vi "getConfigurationConnectionInfo.vi"(8 "error in (no error)":errorcluster, 11 "IDeviceInfo in":refnum<class "IDeviceInfo.lvclass">) -> (0 "error out":errorcluster, 2 "DeviceType out":refnum<class "IServerCapability.lvclass">, 3 "IDeviceInfo out":refnum<class "IDeviceInfo.lvclass">)   [LabVIEW 2022 SP3, in "openDAQ.lvlib" / "IBaseObject.lvlib" / "IPropertyObject.lvlib" / "IDeviceInfo.lvlib" / "IDeviceInfo.lvclass"]
uses:
  <instrlib>/openDAQ/Public/Classes/IDeviceInfo/IDeviceInfo.lvclass
  <instrlib>/openDAQ/Public/Classes/IDeviceInfo/IDeviceInfo.lvclass/IDeviceInfo.ctl
  <instrlib>/openDAQ/Binaries/Windows/x86/copendaq32.dll
  <instrlib>/openDAQ/Public/Classes/IServerCapability/IServerCapability.lvclass
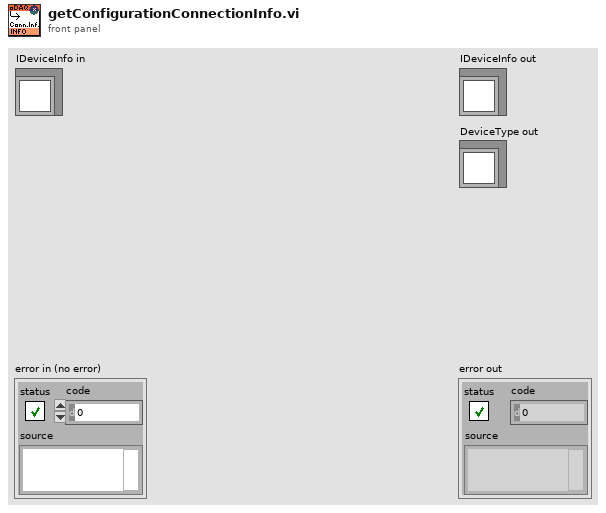
[diagram p1: front panel]
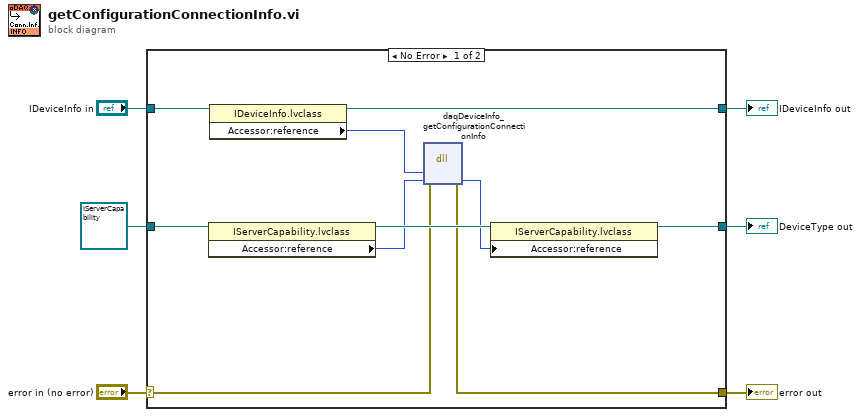
[diagram p0: block diagram]
diagram:
  n1 = case shown="No Error" "error in (no error)" {
    selector: "error in (no error)" -> [w9 w18]
    tunnel: [w7 w18] -> w5
    tunnel: [w13 w17] -> w3
    tunnel: "IDeviceInfo in" -> [w15 w17]
    tunnel: refnum<class "IServerCapability.lvclass"> refnum -> [w10 _]
    tunnel: [w8 _] -> w1
    frame No Error {
      n2 = property class="IServerCapability.lvclass"(reference=w10) -> (reference out=w16:refnum<class "IServerCapability.lvclass">, "Accessor:reference"=w12:i64)  [unwired: 1 in, 1 out]
      n3 = property class="IDeviceInfo.lvclass"(reference=w15) -> (reference out=w13:refnum<class "IDeviceInfo.lvclass">, "Accessor:reference"=w14:i64)  [unwired: 1 in, 1 out]
      n4 = dll-call lib="C:/Program Files (x86)/National Instruments/LabVIEW 2022/instr.lib/openDAQ/Binaries/Windows/x86/copendaq*.*" fn="daqDeviceInfo_getConfigurationConnectionInfo"(error in=w9, "deviceInfo"=w14, "connectionInfo"=w12) -> (error out=w7:errorcluster, "connectionInfo"=w11:i64)  [unwired: 4 in, 1 out]
      n5 = property class="IServerCapability.lvclass"(reference=w16, "Accessor:reference"=w11) -> (reference out=w8:refnum<class "IServerCapability.lvclass">)  [unwired: 1 in, 1 out]
    }
    frame Error {
    }
  }
  "error out" <- w5
  "IDeviceInfo out" <- w3
  "DeviceType out" <- w1
